vi "Spawn Food.vi"(9 "X Position":i32, 10 "Y Position":i32, 11 "Map In":u32[][](array[numeric])) -> (3 "Map Out":u32[][](array[numeric]))   [LabVIEW 2014]
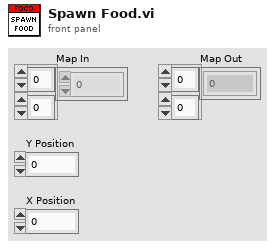
[diagram p1: front panel]
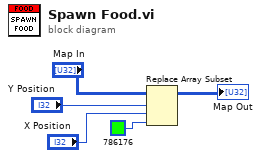
[diagram p0: block diagram]
diagram:
  n1 = Replace Array Subset(array="Map In", new element=u32 786176, index (row)="Y Position", index (col)="X Position") -> (→"Map Out":u32[][])
